vi "Quittieren_SPS.vi"(8 "error in":errorcluster, 11 "Cluster in":T1={"Initialisierung"={"Online?"=FALSE, "Grundpfad"=path "", "Kamera Oben"="", "IP-Adresse Flüssiglinse"="", "Flüssiglinse"=refnum, "Kamera Unten"="", "IP-Adresse SPS"="", "SPS-Verbindung"={"TCP Connection Ref"=refnum, "IP address"="", "timeout ms"=5000, "Connected?"=FALSE, "PLC Type"=enum."S7 1200", "Rack S7 400"=0, "Slot S7 400"=0, "PDU Size"=0, "connection semaphore"=refnum}, "IP-Adresse Lichtgitter"="", "Lichtgitter"=refnum, "Skalierungsfaktor"=0.0, "Bilder Oben"=[], "Bild Unten"=refnum, "Bild Ausschnitt Unten"=refnum}, "Einstellungen"={"Gesamtablauf gestartet"=FALSE, "i. O. Bilder speichern"=FALSE, "Bildspeicherung Offline"=FALSE, "Ausgewähltes Offline-Datum"="", "Ausgewähltes Offline-Teil"="", "Speicherpfad Bilder"=path ""}, "Artikeldaten"={"Artikelnummer"="", "Fertigungsauftrag"="", "Muster ISO"=refnum, "Belichtungszeit Referenzmarken"=0.0, "Fokus Referenzmarken"=0.0, "Belichtungszeit ISO"=0.0, "Fokus ISO"=0.0, "Belichtungszeit Unten"=0.0, "Kontaktanzahl"=0, "Aktueller Kontakt"=0, "Kontaktposition"={"x"=0.0, "y"=0.0}, "ISO-Muster nicht vorhanden"=FALSE, "Winkel ISO"=0.0, "Mittelpunkt ISO"={"x"=0.0, "y"=0.0}}, "Werte Kamera Oben"={"Koordinatensystem"={"Punkt x-Achse"={"X"=0.0, "Y"=0.0}, "Ursprung"={"X"=0.0, "Y"=0.0}, "Punkt y-Achse"={"X"=0.0, "Y"=0.0}}, "Position Kontakt"={"x"=0.0, "y"=0.0}, "Durchmesser Loch"=0.0, "Winkel Kontakt"=0.0, "Position Kontakt umgerechnet"={"x"=0.0, "y"=0.0}}, "Werte Kamera Unten"={"Prüfung Unten n. i. O."=FALSE}, "Werte Lichtgitter"={"Messwerte Referenzmarken"=[], "Mittelpunkt Referenzmarken"={"x"=0.0, "y"=0.0}, "Messwerte Kontakt"=[], "Offset"={"x"=0.0, "y"=0.0}}, "Rückmeldungen"={"Koordinaten ermittelt"=FALSE, "Vermessung Lichtgitter fertig"=FALSE, "Nachkontrolle Kamera Unten fertig"=FALSE}, "Fehler"={"Referenzen nicht gefunden"=FALSE, "Kontakt nicht gefunden"=FALSE, "Referenzen nicht in Lichtgitter"=FALSE, "Kontakt zu groß"=FALSE, "Kontakt zu klein"=FALSE}, "Statistik"={"Statistiken"=[]}, "Timer"={"Timer Start Position"=0, "Timer Start Lichtgitter"=0, "Timer Start Kamera Unten"=0}}) -> (0 "error out":errorcluster, 3 "Cluster out":T1={"Initialisierung"={"Online?"=FALSE, "Grundpfad"=path "", "Kamera Oben"="", "IP-Adresse Flüssiglinse"="", "Flüssiglinse"=refnum, "Kamera Unten"="", "IP-Adresse SPS"="", "SPS-Verbindung"={"TCP Connection Ref"=refnum, "IP address"="", "timeout ms"=5000, "Connected?"=FALSE, "PLC Type"=enum."S7 1200", "Rack S7 400"=0, "Slot S7 400"=0, "PDU Size"=0, "connection semaphore"=refnum}, "IP-Adresse Lichtgitter"="", "Lichtgitter"=refnum, "Skalierungsfaktor"=0.0, "Bilder Oben"=[], "Bild Unten"=refnum, "Bild Ausschnitt Unten"=refnum}, "Einstellungen"={"Gesamtablauf gestartet"=FALSE, "i. O. Bilder speichern"=FALSE, "Bildspeicherung Offline"=FALSE, "Ausgewähltes Offline-Datum"="", "Ausgewähltes Offline-Teil"="", "Speicherpfad Bilder"=path ""}, "Artikeldaten"={"Artikelnummer"="", "Fertigungsauftrag"="", "Muster ISO"=refnum, "Belichtungszeit Referenzmarken"=0.0, "Fokus Referenzmarken"=0.0, "Belichtungszeit ISO"=0.0, "Fokus ISO"=0.0, "Belichtungszeit Unten"=0.0, "Kontaktanzahl"=0, "Aktueller Kontakt"=0, "Kontaktposition"={"x"=0.0, "y"=0.0}, "ISO-Muster nicht vorhanden"=FALSE, "Winkel ISO"=0.0, "Mittelpunkt ISO"={"x"=0.0, "y"=0.0}}, "Werte Kamera Oben"={"Koordinatensystem"={"Punkt x-Achse"={"X"=0.0, "Y"=0.0}, "Ursprung"={"X"=0.0, "Y"=0.0}, "Punkt y-Achse"={"X"=0.0, "Y"=0.0}}, "Position Kontakt"={"x"=0.0, "y"=0.0}, "Durchmesser Loch"=0.0, "Winkel Kontakt"=0.0, "Position Kontakt umgerechnet"={"x"=0.0, "y"=0.0}}, "Werte Kamera Unten"={"Prüfung Unten n. i. O."=FALSE}, "Werte Lichtgitter"={"Messwerte Referenzmarken"=[], "Mittelpunkt Referenzmarken"={"x"=0.0, "y"=0.0}, "Messwerte Kontakt"=[], "Offset"={"x"=0.0, "y"=0.0}}, "Rückmeldungen"={"Koordinaten ermittelt"=FALSE, "Vermessung Lichtgitter fertig"=FALSE, "Nachkontrolle Kamera Unten fertig"=FALSE}, "Fehler"={"Referenzen nicht gefunden"=FALSE, "Kontakt nicht gefunden"=FALSE, "Referenzen nicht in Lichtgitter"=FALSE, "Kontakt zu groß"=FALSE, "Kontakt zu klein"=FALSE}, "Statistik"={"Statistiken"=[]}, "Timer"={"Timer Start Position"=0, "Timer Start Lichtgitter"=0, "Timer Start Kamera Unten"=0}})   [LabVIEW 2024]
uses:
  Typdefinitionen/Cluster.ctl
  <vilib>/userDefined/High Color/IMAQdx.ctl
  <vilib>/DATA AHEAD/SP7/typedefs/S7 Connection.ctl
  <vilib>/DATA AHEAD/SP7/typedefs/PLC Type.ctl
  <vilib>/vision/Image Controls.llb/IMAQ Image.ctl
  Typdefinitionen/Koordinatensystem.ctl
  Typdefinitionen/Statistik.ctl
  Sonstige/Globale Variablen.vi
  <vilib>/DATA AHEAD/SP7/functions/write/write bool array.vi
  <vilib>/DATA AHEAD/SP7/SP7.lvlib
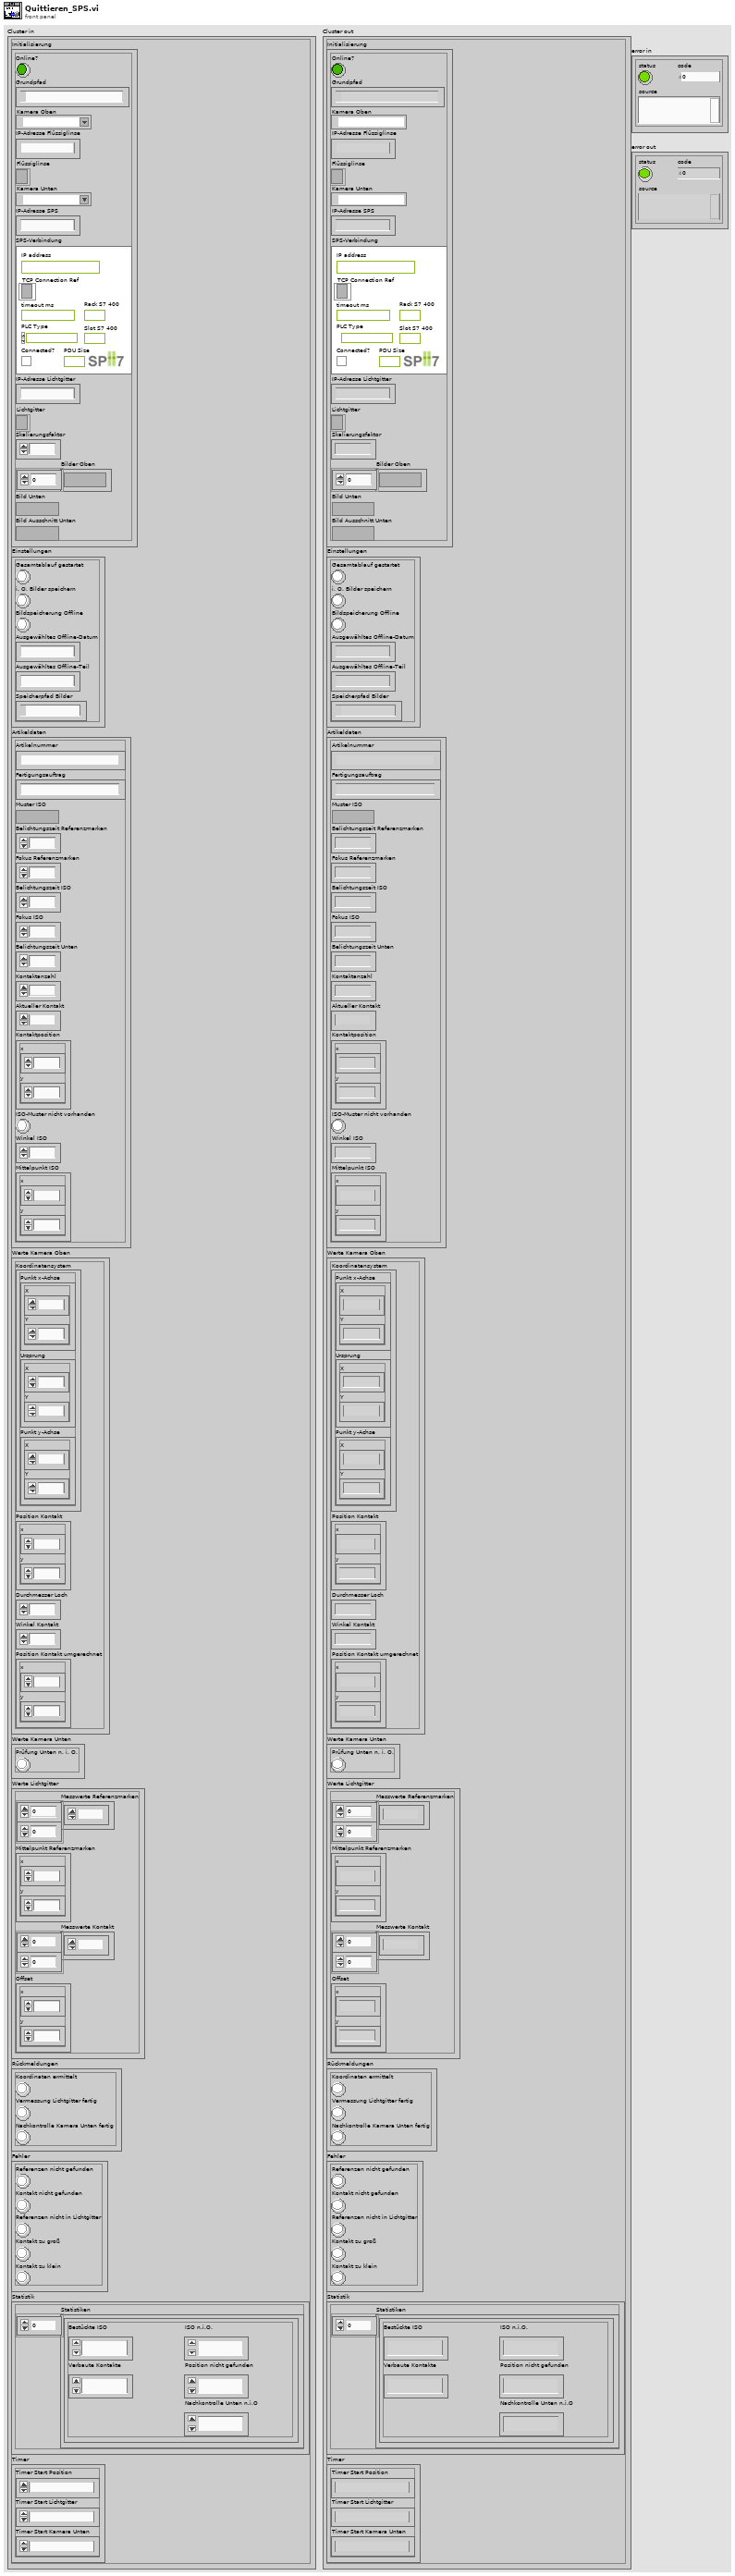
[diagram p1: front panel]
types:
  T1 = typedef "Cluster.ctl" = cluster{"Initialisierung":cluster{"Online?":bool, "Grundpfad":path, "Kamera Oben":T2, "IP-Adresse Flüssiglinse":string, "Flüssiglinse":refnum<k5>, "Kamera Unten":T2, "IP-Adresse SPS":string, "SPS-Verbindung":T3, "IP-Adresse Lichtgitter":string, "Lichtgitter":refnum<k5>, "Skalierungsfaktor":dbl, "Bilder Oben":T6[], "Bild Unten":T6, "Bild Ausschnitt Unten":T6}, "Einstellungen":cluster{"Gesamtablauf gestartet":bool, "i. O. Bilder speichern":bool, "Bildspeicherung Offline":bool, "Ausgewähltes Offline-Datum":string, "Ausgewähltes Offline-Teil":string, "Speicherpfad Bilder":path}, "Artikeldaten":cluster{"Artikelnummer":string, "Fertigungsauftrag":string, "Muster ISO":T6, "Belichtungszeit Referenzmarken":dbl, "Fokus Referenzmarken":dbl, "Belichtungszeit ISO":dbl, "Fokus ISO":dbl, "Belichtungszeit Unten":dbl, "Kontaktanzahl":u32, "Aktueller Kontakt":i16, "Kontaktposition":cluster{"x":sgl, "y":sgl}, "ISO-Muster nicht vorhanden":bool, "Winkel ISO":sgl, "Mittelpunkt ISO":cluster{"x":dbl, "y":dbl}}, "Werte Kamera Oben":cluster{"Koordinatensystem":T7, "Position Kontakt":cluster{"x":dbl, "y":dbl}, "Durchmesser Loch":dbl, "Winkel Kontakt":dbl, "Position Kontakt umgerechnet":cluster{"x":dbl, "y":dbl}}, "Werte Kamera Unten":cluster{"Prüfung Unten n. i. O.":bool}, "Werte Lichtgitter":cluster{"Messwerte Referenzmarken":dbl[][], "Mittelpunkt Referenzmarken":cluster{"x":dbl, "y":dbl}, "Messwerte Kontakt":dbl[][], "Offset":cluster{"x":dbl, "y":dbl}}, "Rückmeldungen":cluster{"Koordinaten ermittelt":bool, "Vermessung Lichtgitter fertig":bool, "Nachkontrolle Kamera Unten fertig":bool}, "Fehler":cluster{"Referenzen nicht gefunden":bool, "Kontakt nicht gefunden":bool, "Referenzen nicht in Lichtgitter":bool, "Kontakt zu groß":bool, "Kontakt zu klein":bool}, "Statistik":cluster{"Statistiken":T8[]}, "Timer":cluster{"Timer Start Position":u32, "Timer Start Lichtgitter":u32, "Timer Start Kamera Unten":u32}}
  T2 = typedef "IMAQdx.ctl" = refnum<k21>
  T3 = typedef "SP7.lvlib/S7 Connection.ctl" = cluster{"TCP Connection Ref":refnum<k5>, "IP address":string, "timeout ms":i32, "Connected?":bool, "PLC Type":T4, "Rack S7 400":u8, "Slot S7 400":u8, "PDU Size":u16, "connection semaphore":T5}
  T4 = typedef "SP7.lvlib/PLC Type.ctl" = enum16{"S7 200", "S7 300/400", "S7 1200", "S7 1500", "LOGO!8"}
  T5 = typedef "Semaphore RefNum" = refnum<k1>
  T6 = typedef "IMAQ Image.ctl" = refnum<image>
  T7 = typedef "Koordinatensystem.ctl" = cluster{"Punkt x-Achse":cluster{"X":sgl, "Y":sgl}, "Ursprung":cluster{"X":sgl, "Y":sgl}, "Punkt y-Achse":cluster{"X":sgl, "Y":sgl}}
  T8 = typedef "Statistik.ctl" = cluster{"Bestückte ISO":u32, "Verbaute Kontakte":u32, "ISO n.i.O.":u32, "Nachkontrolle Unten n.i.O":u32, "Position nicht gefunden":u32}
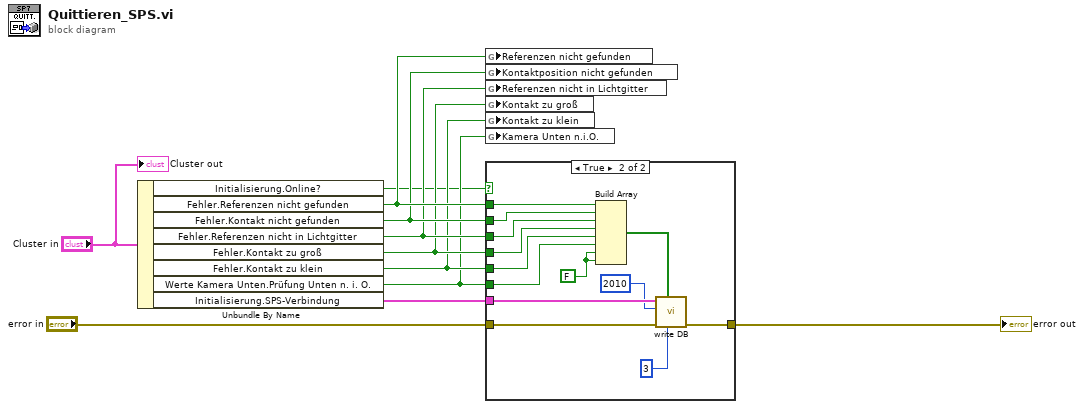
[diagram p0: block diagram]
diagram:
  n1 = Unbundle By Name("Cluster in") -> ("Initialisierung.Online?"=w1:bool, "Fehler.Referenzen nicht gefunden"=w7:bool, "Fehler.Kontakt nicht gefunden"=w6:bool, "Fehler.Referenzen nicht in Lichtgitter"=w5:bool, "Fehler.Kontakt zu groß"=w4:bool, "Fehler.Kontakt zu klein"=w3:bool, "Werte Kamera Unten.Prüfung Unten n. i. O."=w2:bool, "Initialisierung.SPS-Verbindung"=w11:T3)
  n2 = global write "Globale Variablen.vi" "Referenzen nicht gefunden"(w7) -> ()
  n3 = global write "Globale Variablen.vi" "Kontaktposition nicht gefunden"(w6) -> ()
  n4 = global write "Globale Variablen.vi" "Referenzen nicht in Lichtgitter"(w5) -> ()
  n5 = global write "Globale Variablen.vi" "Kontakt zu groß"(w4) -> ()
  n6 = global write "Globale Variablen.vi" "Kontakt zu klein"(w3) -> ()
  n7 = global write "Globale Variablen.vi" "Kamera Unten n.i.O."(w2) -> ()
  n8 = case shown="True" w1 {
    tunnel: w11 -> [_ w25]
    tunnel: [w12 w21] -> w9
    tunnel: "error in" -> [w12 w24]
    tunnel: w7 -> [_ w20]
    tunnel: w6 -> [_ w19]
    tunnel: w5 -> [_ w18]
    tunnel: w4 -> [_ w17]
    tunnel: w3 -> [_ w16]
    tunnel: w2 -> [_ w13]
    frame False {
    }
    frame True {
      w15 = FALSE
      n9 = Build Array(w20, w19, w18, w17, w16, w13, w15, w15) -> (w23:bool[])
      n10 = call-poly <vilib>:"write DB.vi"("Item offset [byte]"=u32 3, "BOOL input array [byte]"=w23, "error in (no error)"=w24, "Data Block #"=u16 2010, "S7 Connection in"=w25) -> ("error out"=w21:errorcluster)  [unwired: 3 in, 3 out]
    }
  }
  "error out" <- w9
  "Cluster out" <- "Cluster in"
